vi "WILT Injection Timer 2.vi"(4 "Injection Times":T1, 7 "Station Number in":u32, 8 "Error In":errorcluster, 9 "Current Threshold":dbl=1.0 format="%#_13g", 10 "Step 3 Input":T3, 11 "Dryer Step Pause In":T5 {"Night Cycle Count" format="%04d"; "Day Cycle Count" format="%04d"}) -> (0 "Error Out":errorcluster, 2 "Step 5 Output":T3, 3 "Dryer Step Pause Output":T5 {"Night Cycle Count" format="%04d"; "Day Cycle Count" format="%04d"})   [LabVIEW 2016]
uses:
  Type Definitions/WILT Station Test State Cluster.ctl
  Type Definitions/WILT Dryer Test State.ctl
  Type Definitions/WILT Dryer.ctl
  Type Definitions/WILT Dryer Details.ctl
  Type Definitions/WILT Agilent Channel Definition.ctl
  Type Definitions/WILT DAQ Data.ctl
  Type Definitions/WILT Injection Times.ctl
  Type Definitions/WILT Water Injection Control.ctl
  Globals/WILT Globals Main Program.vi
panel:
  # "Day"
  # "Night"
  # "Day"
  # "Night"
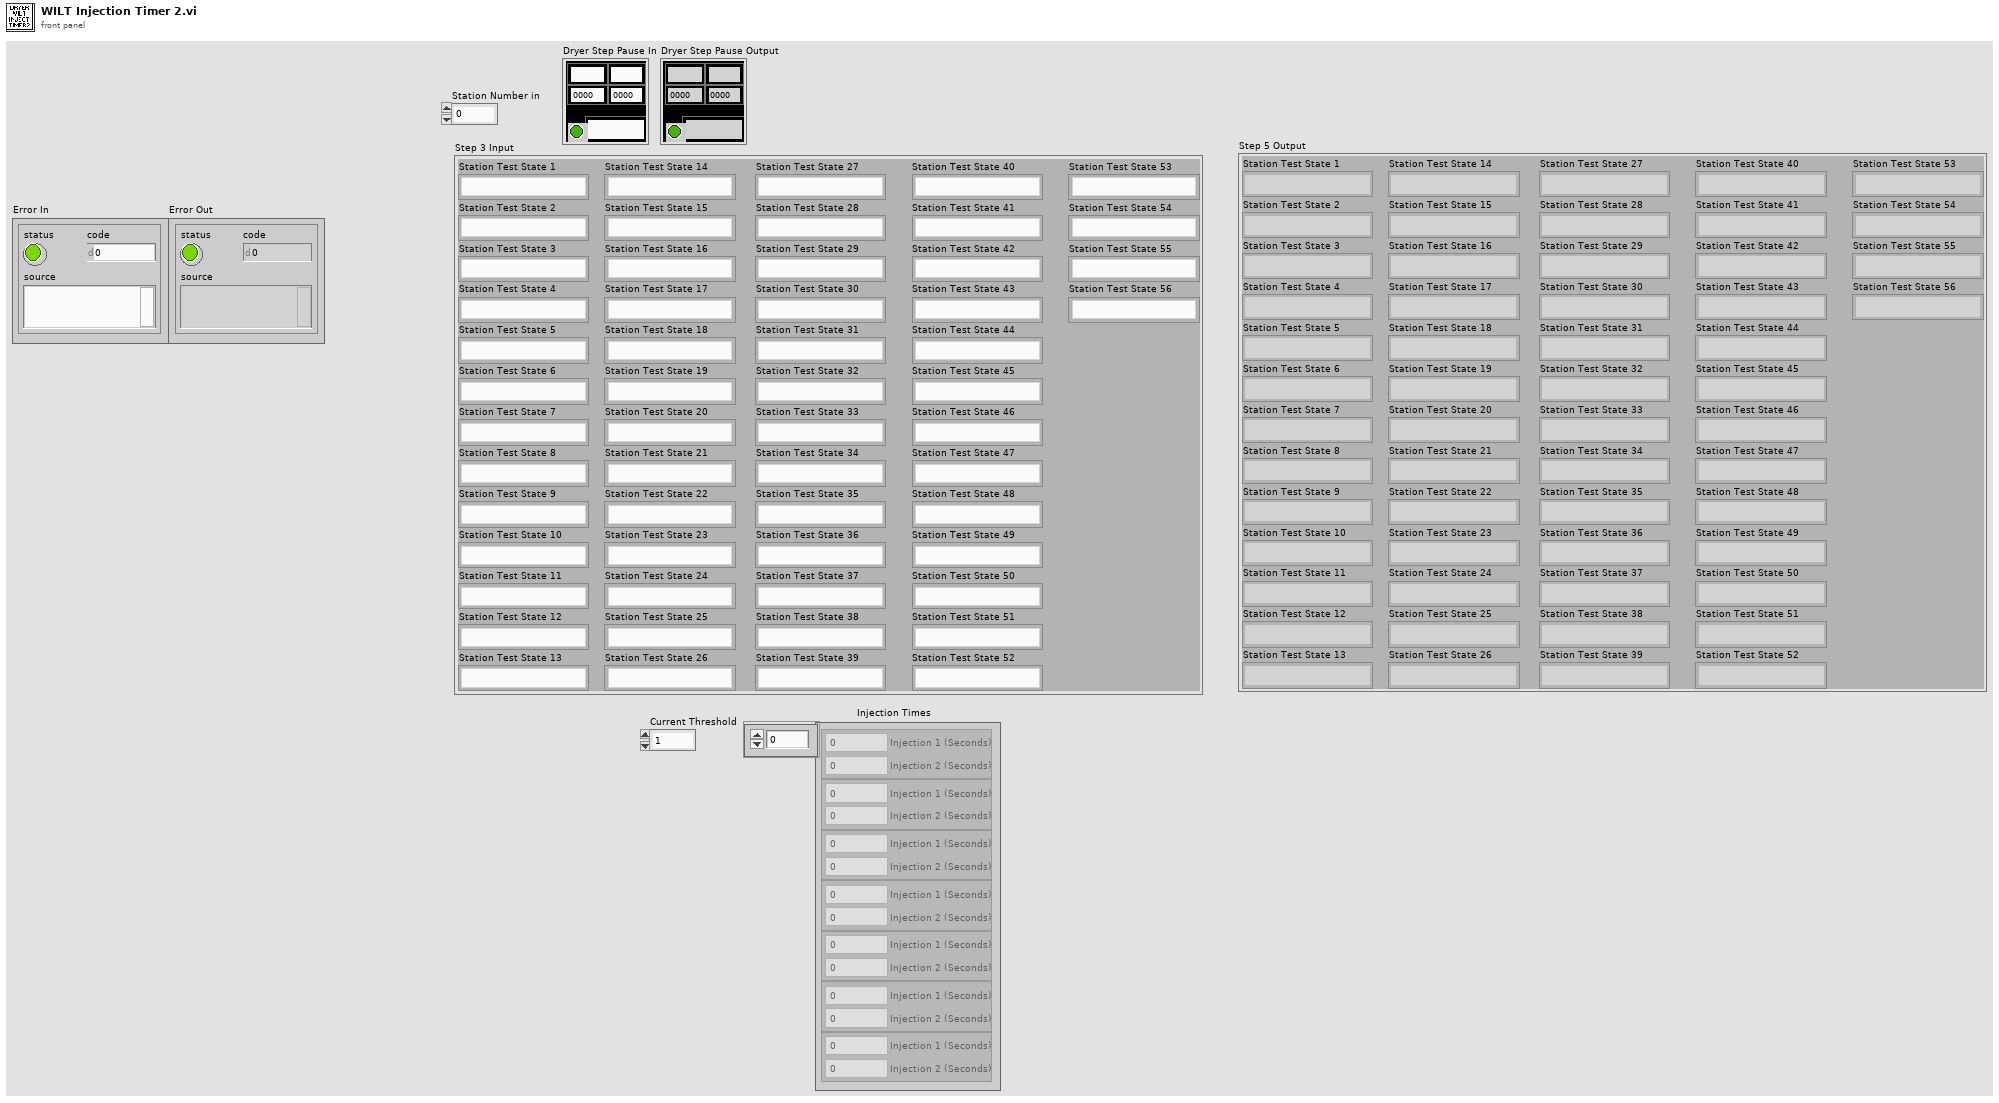
[diagram p1: front panel]
types:
  T1 = typedef "WILT Injection Times.ctl" = T2[]
  T2 = typedef "WILT Water Injection Control.ctl" = cluster{"Injection 1 (Seconds)":dbl, "Injection 2 (Seconds)":dbl}
  T3 = typedef "WILT Station Test State Cluster.ctl" = cluster{"Station Test State 1":T4, "Station Test State 2":T4, "Station Test State 3":T4, "Station Test State 4":T4, "Station Test State 5":T4, "Station Test State 6":T4, "Station Test State 7":T4, "Station Test State 8":T4, "Station Test State 9":T4, "Station Test State 10":T4, "Station Test State 11":T4, "Station Test State 12":T4, "Station Test State 13":T4, "Station Test State 14":T4, "Station Test State 15":T4, "Station Test State 16":T4, "Station Test State 17":T4, "Station Test State 18":T4, "Station Test State 19":T4, "Station Test State 20":T4, "Station Test State 21":T4, "Station Test State 22":T4, "Station Test State 23":T4, "Station Test State 24":T4, "Station Test State 25":T4, "Station Test State 26":T4, "Station Test State 27":T4, "Station Test State 28":T4, "Station Test State 29":T4, "Station Test State 30":T4, "Station Test State 31":T4, "Station Test State 32":T4, "Station Test State 33":T4, "Station Test State 34":T4, "Station Test State 35":T4, "Station Test State 36":T4, "Station Test State 37":T4, "Station Test State 38":T4, "Station Test State 39":T4, "Station Test State 40":T4, "Station Test State 41":T4, "Station Test State 42":T4, "Station Test State 43":T4, "Station Test State 44":T4, "Station Test State 45":T4, "Station Test State 46":T4, "Station Test State 47":T4, "Station Test State 48":T4, "Station Test State 49":T4, "Station Test State 50":T4, "Station Test State 51":T4, "Station Test State 52":T4, "Station Test State 53":T4, "Station Test State 54":T4, "Station Test State 55":T4, "Station Test State 56":T4}
  T4 = typedef "WILT Dryer Test State.ctl" = enum16{"No Serial Number", "Waiting for Dryer To Start", "Drying Clothes", "Water Injection 1 (On)", "Water Injection 1 Timer", "Water Injection 1 (Off)", "Pause Dryer", "Sending Start Stop CMD", "Pause Dryer 2", "Sending Start Stop CMD 2", "Drying Clothes 2", "Water Injection 2 (On)", "Water Injection 2 Timer", "Water Injection 2 (Off)", "Drying Clothes 3", "Cooling Down", "Sending Start Stop CMD 3", "Increment Cycle"}
  T5 = typedef "WILT Dryer.ctl" = cluster{"Lab ID":string, "Day Cycle Count":i32, "Station Label":string, "Dryer Details":T6, "Status Color":u32, "Invisible Button":bool, "Night Cycle Count":i32, "Station Index":i32, "Cycle Index":string, "Audit Alert":bool, "Agilent Channel Definition":T7, "DAQ Data":T8}
  T6 = typedef "WILT Dryer Details.ctl" = cluster{"Station":string, "Lab ID":string, "TR Number":string}
  T7 = typedef "WILT Agilent Channel Definition.ctl" = cluster{"Channel":string, "Station":string, "Label":string, "Agilent Station":string, "Data":dbl}
  T8 = typedef "WILT DAQ Data.ctl" = cluster{"L1 Current":dbl, "L2 Current":dbl, "Temperature  Deg F (TC)":dbl, "Volts":dbl, "Volts (208)":dbl, "SW (208)":dbl}
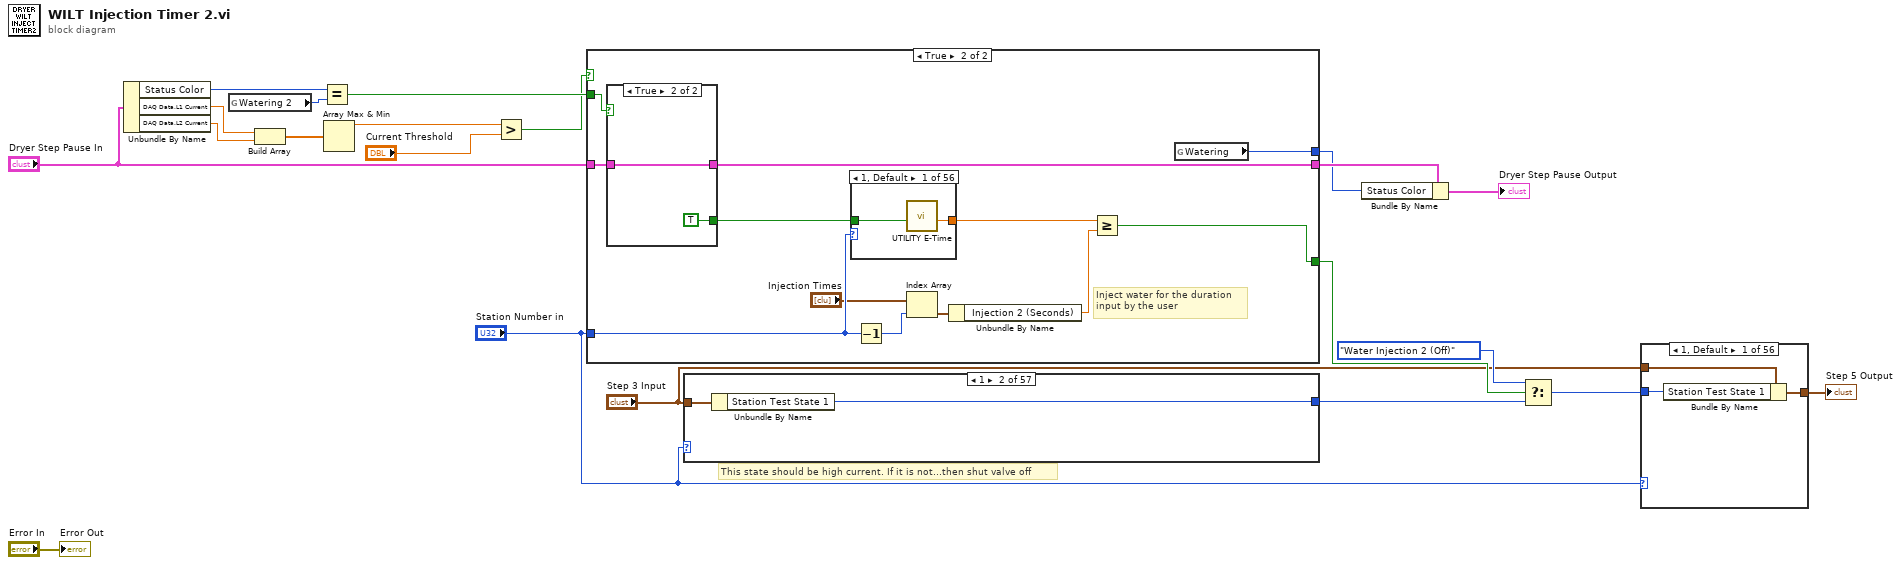
[diagram p0: block diagram]
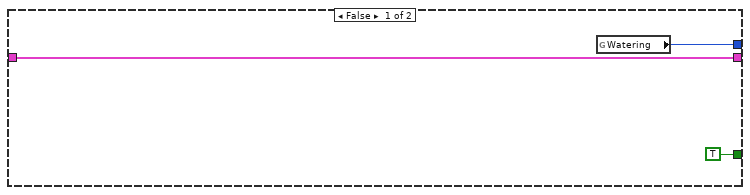
[diagram p2: hidden frame]
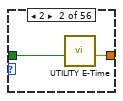
[diagram p3: hidden frame]
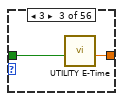
[diagram p4: hidden frame]
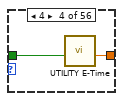
[diagram p5: hidden frame]
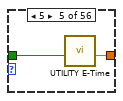
[diagram p6: hidden frame]
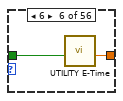
[diagram p7: hidden frame]
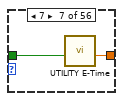
[diagram p8: hidden frame]
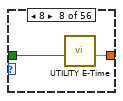
[diagram p9: hidden frame]
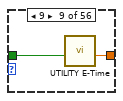
[diagram p10: hidden frame]
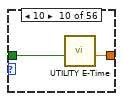
[diagram p11: hidden frame]
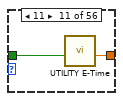
[diagram p12: hidden frame]
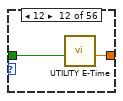
[diagram p13: hidden frame]
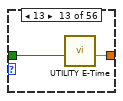
[diagram p14: hidden frame]
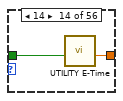
[diagram p15: hidden frame]
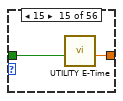
[diagram p16: hidden frame]
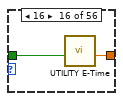
[diagram p17: hidden frame]
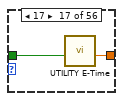
[diagram p18: hidden frame]
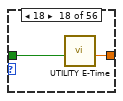
[diagram p19: hidden frame]
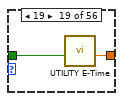
[diagram p20: hidden frame]
diagram:
  # "This state should be high current. If it is not...then shut valve off"
  n1 = Unbundle By Name("Dryer Step Pause In") -> ("Status Color"=w14:u32, "DAQ Data.L1 Current"=w7:dbl, "DAQ Data.L2 Current"=w6:dbl)
  n2 = global read "WILT Globals Main Program.vi" "Watering 2"() -> (w10:u32)
  n3 = Build Array(w7, w6) -> (w5:dbl[])
  n4 = Equal?(x=w14, y=w10) -> (x = y?=w9:bool)
  n5 = Array Max & Min(array=w5) -> (max value=w4:dbl)  [unwired: 3 out]
  n6 = Greater?(x=w4, y="Current Threshold") -> (0:w2:bool)
  n7 = case shown="True" w2 {
    tunnel: [TRUE w36] -> w20
    tunnel: "Dryer Step Pause In" -> [w24 w34]
    tunnel: "Station Number in" -> [_ w33]
    tunnel: w9 -> [_ w30]
    tunnel: [w24 w29] -> w8
    tunnel: [w23 w25] -> w1
    frame False {
      n8 = global read "WILT Globals Main Program.vi" "Watering"() -> (w23:u32)
    }
    frame True {
      # "Inject water for the duration \ninput by the user"
      n9 = case shown="True" w30 {
        tunnel: [FALSE TRUE] -> w28
        tunnel: w34 -> [w149 w151]
        tunnel: [w149 w151] -> w29
        frame False {
        }
        frame True {
        }
      }
      n10 = case shown="1, Default" w33 {
        tunnel: [w38 w39 w41 w43 w45 w47 w49 w51 w53 w55 w57 w59 w61 w63 w65 w67 w69 w71 w73 w75 w77 w79 w81 w83 w85 w87 w89 w91 w93 w95 w97 w99 w101 w103 w105 w107 w109 w111 w113 w115 w117 w119 w121 w123 w125 w127 w129 w131 w133 w135 w137 w139 w141 w143 w145 w147] -> w27
        tunnel: w28 -> [w37 w40 w42 w44 w46 w48 w50 w52 w54 w56 w58 w60 w62 w64 w66 w68 w70 w72 w74 w76 w78 w80 w82 w84 w86 w88 w90 w92 w94 w96 w98 w100 w102 w104 w106 w108 w110 w112 w114 w116 w118 w120 w122 w124 w126 w128 w130 w132 w134 w136 w138 w140 w142 w144 w146 w148]
        frame 1, Default {
          n11 = call "UTILITY E-Time.vi"("Reset"=w37) -> ("Elapsed Time (sec)"=w38:dbl)  [unwired: 8 in, 2 out]
        }
        frame 2 {
          n12 = call "UTILITY E-Time.vi"("Reset"=w40) -> ("Elapsed Time (sec)"=w39:dbl)  [unwired: 8 in, 2 out]
        }
        frame 3 {
          n13 = call "UTILITY E-Time.vi"("Reset"=w42) -> ("Elapsed Time (sec)"=w41:dbl)  [unwired: 8 in, 2 out]
        }
        frame 4 {
          n14 = call "UTILITY E-Time.vi"("Reset"=w44) -> ("Elapsed Time (sec)"=w43:dbl)  [unwired: 8 in, 2 out]
        }
        frame 5 {
          n15 = call "UTILITY E-Time.vi"("Reset"=w46) -> ("Elapsed Time (sec)"=w45:dbl)  [unwired: 8 in, 2 out]
        }
        frame 6 {
          n16 = call "UTILITY E-Time.vi"("Reset"=w48) -> ("Elapsed Time (sec)"=w47:dbl)  [unwired: 8 in, 2 out]
        }
        frame 7 {
          n17 = call "UTILITY E-Time.vi"("Reset"=w50) -> ("Elapsed Time (sec)"=w49:dbl)  [unwired: 8 in, 2 out]
        }
        frame 8 {
          n18 = call "UTILITY E-Time.vi"("Reset"=w52) -> ("Elapsed Time (sec)"=w51:dbl)  [unwired: 8 in, 2 out]
        }
        frame 9 {
          n19 = call "UTILITY E-Time.vi"("Reset"=w54) -> ("Elapsed Time (sec)"=w53:dbl)  [unwired: 8 in, 2 out]
        }
        frame 10 {
          n20 = call "UTILITY E-Time.vi"("Reset"=w56) -> ("Elapsed Time (sec)"=w55:dbl)  [unwired: 8 in, 2 out]
        }
        frame 11 {
          n21 = call "UTILITY E-Time.vi"("Reset"=w58) -> ("Elapsed Time (sec)"=w57:dbl)  [unwired: 8 in, 2 out]
        }
        frame 12 {
          n22 = call "UTILITY E-Time.vi"("Reset"=w60) -> ("Elapsed Time (sec)"=w59:dbl)  [unwired: 8 in, 2 out]
        }
        frame 13 {
          n23 = call "UTILITY E-Time.vi"("Reset"=w62) -> ("Elapsed Time (sec)"=w61:dbl)  [unwired: 8 in, 2 out]
        }
        frame 14 {
          n24 = call "UTILITY E-Time.vi"("Reset"=w64) -> ("Elapsed Time (sec)"=w63:dbl)  [unwired: 8 in, 2 out]
        }
        frame 15 {
          n25 = call "UTILITY E-Time.vi"("Reset"=w66) -> ("Elapsed Time (sec)"=w65:dbl)  [unwired: 8 in, 2 out]
        }
        frame 16 {
          n26 = call "UTILITY E-Time.vi"("Reset"=w68) -> ("Elapsed Time (sec)"=w67:dbl)  [unwired: 8 in, 2 out]
        }
        frame 17 {
          n27 = call "UTILITY E-Time.vi"("Reset"=w70) -> ("Elapsed Time (sec)"=w69:dbl)  [unwired: 8 in, 2 out]
        }
        frame 18 {
          n28 = call "UTILITY E-Time.vi"("Reset"=w72) -> ("Elapsed Time (sec)"=w71:dbl)  [unwired: 8 in, 2 out]
        }
        frame 19 {
          n29 = call "UTILITY E-Time.vi"("Reset"=w74) -> ("Elapsed Time (sec)"=w73:dbl)  [unwired: 8 in, 2 out]
        }
        frame 20 {
          n30 = call "UTILITY E-Time.vi"("Reset"=w76) -> ("Elapsed Time (sec)"=w75:dbl)  [unwired: 8 in, 2 out]
        }
        frame 21 {
          n31 = call "UTILITY E-Time.vi"("Reset"=w78) -> ("Elapsed Time (sec)"=w77:dbl)  [unwired: 8 in, 2 out]
        }
        frame 22 {
          n32 = call "UTILITY E-Time.vi"("Reset"=w80) -> ("Elapsed Time (sec)"=w79:dbl)  [unwired: 8 in, 2 out]
        }
        frame 23 {
          n33 = call "UTILITY E-Time.vi"("Reset"=w82) -> ("Elapsed Time (sec)"=w81:dbl)  [unwired: 8 in, 2 out]
        }
        frame 24 {
          n34 = call "UTILITY E-Time.vi"("Reset"=w84) -> ("Elapsed Time (sec)"=w83:dbl)  [unwired: 8 in, 2 out]
        }
        frame 25 {
          n35 = call "UTILITY E-Time.vi"("Reset"=w86) -> ("Elapsed Time (sec)"=w85:dbl)  [unwired: 8 in, 2 out]
        }
        frame 26 {
          n36 = call "UTILITY E-Time.vi"("Reset"=w88) -> ("Elapsed Time (sec)"=w87:dbl)  [unwired: 8 in, 2 out]
        }
        frame 27 {
          n37 = call "UTILITY E-Time.vi"("Reset"=w90) -> ("Elapsed Time (sec)"=w89:dbl)  [unwired: 8 in, 2 out]
        }
        frame 28 {
          n38 = call "UTILITY E-Time.vi"("Reset"=w92) -> ("Elapsed Time (sec)"=w91:dbl)  [unwired: 8 in, 2 out]
        }
        frame 29 {
          n39 = call "UTILITY E-Time.vi"("Reset"=w94) -> ("Elapsed Time (sec)"=w93:dbl)  [unwired: 8 in, 2 out]
        }
        frame 30 {
          n40 = call "UTILITY E-Time.vi"("Reset"=w96) -> ("Elapsed Time (sec)"=w95:dbl)  [unwired: 8 in, 2 out]
        }
        frame 31 {
          n41 = call "UTILITY E-Time.vi"("Reset"=w98) -> ("Elapsed Time (sec)"=w97:dbl)  [unwired: 8 in, 2 out]
        }
        frame 32 {
          n42 = call "UTILITY E-Time.vi"("Reset"=w100) -> ("Elapsed Time (sec)"=w99:dbl)  [unwired: 8 in, 2 out]
        }
        frame 33 {
          n43 = call "UTILITY E-Time.vi"("Reset"=w102) -> ("Elapsed Time (sec)"=w101:dbl)  [unwired: 8 in, 2 out]
        }
        frame 34 {
          n44 = call "UTILITY E-Time.vi"("Reset"=w104) -> ("Elapsed Time (sec)"=w103:dbl)  [unwired: 8 in, 2 out]
        }
        frame 35 {
          n45 = call "UTILITY E-Time.vi"("Reset"=w106) -> ("Elapsed Time (sec)"=w105:dbl)  [unwired: 8 in, 2 out]
        }
        frame 36 {
          n46 = call "UTILITY E-Time.vi"("Reset"=w108) -> ("Elapsed Time (sec)"=w107:dbl)  [unwired: 8 in, 2 out]
        }
        frame 37 {
          n47 = call "UTILITY E-Time.vi"("Reset"=w110) -> ("Elapsed Time (sec)"=w109:dbl)  [unwired: 8 in, 2 out]
        }
        frame 38 {
          n48 = call "UTILITY E-Time.vi"("Reset"=w112) -> ("Elapsed Time (sec)"=w111:dbl)  [unwired: 8 in, 2 out]
        }
        frame 39 {
          n49 = call "UTILITY E-Time.vi"("Reset"=w114) -> ("Elapsed Time (sec)"=w113:dbl)  [unwired: 8 in, 2 out]
        }
        frame 40 {
          n50 = call "UTILITY E-Time.vi"("Reset"=w116) -> ("Elapsed Time (sec)"=w115:dbl)  [unwired: 8 in, 2 out]
        }
        frame 41 {
          n51 = call "UTILITY E-Time.vi"("Reset"=w118) -> ("Elapsed Time (sec)"=w117:dbl)  [unwired: 8 in, 2 out]
        }
        frame 42 {
          n52 = call "UTILITY E-Time.vi"("Reset"=w120) -> ("Elapsed Time (sec)"=w119:dbl)  [unwired: 8 in, 2 out]
        }
        frame 43 {
          n53 = call "UTILITY E-Time.vi"("Reset"=w122) -> ("Elapsed Time (sec)"=w121:dbl)  [unwired: 8 in, 2 out]
        }
        frame 44 {
          n54 = call "UTILITY E-Time.vi"("Reset"=w124) -> ("Elapsed Time (sec)"=w123:dbl)  [unwired: 8 in, 2 out]
        }
        frame 45 {
          n55 = call "UTILITY E-Time.vi"("Reset"=w126) -> ("Elapsed Time (sec)"=w125:dbl)  [unwired: 8 in, 2 out]
        }
        frame 46 {
          n56 = call "UTILITY E-Time.vi"("Reset"=w128) -> ("Elapsed Time (sec)"=w127:dbl)  [unwired: 8 in, 2 out]
        }
        frame 47 {
          n57 = call "UTILITY E-Time.vi"("Reset"=w130) -> ("Elapsed Time (sec)"=w129:dbl)  [unwired: 8 in, 2 out]
        }
        frame 48 {
          n58 = call "UTILITY E-Time.vi"("Reset"=w132) -> ("Elapsed Time (sec)"=w131:dbl)  [unwired: 8 in, 2 out]
        }
        frame 49 {
          n59 = call "UTILITY E-Time.vi"("Reset"=w134) -> ("Elapsed Time (sec)"=w133:dbl)  [unwired: 8 in, 2 out]
        }
        frame 50 {
          n60 = call "UTILITY E-Time.vi"("Reset"=w136) -> ("Elapsed Time (sec)"=w135:dbl)  [unwired: 8 in, 2 out]
        }
        frame 51 {
          n61 = call "UTILITY E-Time.vi"("Reset"=w138) -> ("Elapsed Time (sec)"=w137:dbl)  [unwired: 8 in, 2 out]
        }
        frame 52 {
          n62 = call "UTILITY E-Time.vi"("Reset"=w140) -> ("Elapsed Time (sec)"=w139:dbl)  [unwired: 8 in, 2 out]
        }
        frame 53 {
          n63 = call "UTILITY E-Time.vi"("Reset"=w142) -> ("Elapsed Time (sec)"=w141:dbl)  [unwired: 8 in, 2 out]
        }
        frame 54 {
          n64 = call "UTILITY E-Time.vi"("Reset"=w144) -> ("Elapsed Time (sec)"=w143:dbl)  [unwired: 8 in, 2 out]
        }
        frame 55 {
          n65 = call "UTILITY E-Time.vi"("Reset"=w146) -> ("Elapsed Time (sec)"=w145:dbl)  [unwired: 8 in, 2 out]
        }
        frame 56 {
          n66 = call "UTILITY E-Time.vi"("Reset"=w148) -> ("Elapsed Time (sec)"=w147:dbl)  [unwired: 8 in, 2 out]
        }
      }
      n67 = Decrement(x=w33) -> (x-1=w35:u32)
      n68 = Index Array(array="Injection Times", index=w35) -> (element=w32:T2)
      n69 = Unbundle By Name(w32) -> ("Injection 2 (Seconds)"=w31:dbl)
      n70 = Greater Or Equal?(x=w27, y=w31) -> (x >= y?=w36:bool)
      n71 = global read "WILT Globals Main Program.vi" "Watering"() -> (w25:u32)
    }
  }
  n72 = case shown="1" "Station Number in" {
    tunnel: "Step 3 Input" -> [_ w155 w157 w159 w161 w163 w165 w167 w169 w171 w173 w175 w177 w179 w181 w183 w185 w187 w189 w191 w193 w195 w197 w199 w201 w203 w205 w207 w209 w211 w213 w215 w217 w219 w221 w223 w225 w227 w229 w231 w233 w235 w237 w239 w241 w243 w245 w247 w249 w251 w253 w255 w257 w259 w261 w263 w265]
    tunnel: [WILT_Dryer_Test_State."No Serial Number" ("Station Test State 56") w154 w156 w158 w160 w162 w164 w166 w168 w170 w172 w174 w176 w178 w180 w182 w184 w186 w188 w190 w192 w194 w196 w198 w200 w202 w204 w206 w208 w210 w212 w214 w216 w218 w220 w222 w224 w226 w228 w230 w232 w234 w236 w238 w240 w242 w244 w246 w248 w250 w252 w254 w256 w258 w260 w262 w264] -> w16
    frame 0, Default {
      # "This is not a station.\nDo nothing"
    }
    frame 1 {
      n73 = Unbundle By Name(w155) -> ("Station Test State 1"=w154:T4)
    }
    frame 2 {
      n74 = Unbundle By Name(w157) -> ("Station Test State 2"=w156:T4)
    }
    frame 3 {
      n75 = Unbundle By Name(w159) -> ("Station Test State 3"=w158:T4)
    }
    frame 4 {
      n76 = Unbundle By Name(w161) -> ("Station Test State 4"=w160:T4)
    }
    frame 5 {
      n77 = Unbundle By Name(w163) -> ("Station Test State 5"=w162:T4)
    }
    frame 6 {
      n78 = Unbundle By Name(w165) -> ("Station Test State 6"=w164:T4)
    }
    frame 7 {
      n79 = Unbundle By Name(w167) -> ("Station Test State 7"=w166:T4)
    }
    frame 8 {
      n80 = Unbundle By Name(w169) -> ("Station Test State 8"=w168:T4)
    }
    frame 9 {
      n81 = Unbundle By Name(w171) -> ("Station Test State 9"=w170:T4)
    }
    frame 10 {
      n82 = Unbundle By Name(w173) -> ("Station Test State 10"=w172:T4)
    }
    frame 11 {
      n83 = Unbundle By Name(w175) -> ("Station Test State 11"=w174:T4)
    }
    frame 12 {
      n84 = Unbundle By Name(w177) -> ("Station Test State 12"=w176:T4)
    }
    frame 13 {
      n85 = Unbundle By Name(w179) -> ("Station Test State 13"=w178:T4)
    }
    frame 14 {
      n86 = Unbundle By Name(w181) -> ("Station Test State 14"=w180:T4)
    }
    frame 15 {
      n87 = Unbundle By Name(w183) -> ("Station Test State 15"=w182:T4)
    }
    frame 16 {
      n88 = Unbundle By Name(w185) -> ("Station Test State 16"=w184:T4)
    }
    frame 17 {
      n89 = Unbundle By Name(w187) -> ("Station Test State 17"=w186:T4)
    }
    frame 18 {
      n90 = Unbundle By Name(w189) -> ("Station Test State 18"=w188:T4)
    }
    frame 19 {
      n91 = Unbundle By Name(w191) -> ("Station Test State 19"=w190:T4)
    }
    frame 20 {
      n92 = Unbundle By Name(w193) -> ("Station Test State 20"=w192:T4)
    }
    frame 21 {
      n93 = Unbundle By Name(w195) -> ("Station Test State 21"=w194:T4)
    }
    frame 22 {
      n94 = Unbundle By Name(w197) -> ("Station Test State 22"=w196:T4)
    }
    frame 23 {
      n95 = Unbundle By Name(w199) -> ("Station Test State 23"=w198:T4)
    }
    frame 24 {
      n96 = Unbundle By Name(w201) -> ("Station Test State 24"=w200:T4)
    }
    frame 25 {
      n97 = Unbundle By Name(w203) -> ("Station Test State 25"=w202:T4)
    }
    frame 26 {
      n98 = Unbundle By Name(w205) -> ("Station Test State 26"=w204:T4)
    }
    frame 27 {
      n99 = Unbundle By Name(w207) -> ("Station Test State 27"=w206:T4)
    }
    frame 28 {
      n100 = Unbundle By Name(w209) -> ("Station Test State 28"=w208:T4)
    }
    frame 29 {
      n101 = Unbundle By Name(w211) -> ("Station Test State 29"=w210:T4)
    }
    frame 30 {
      n102 = Unbundle By Name(w213) -> ("Station Test State 30"=w212:T4)
    }
    frame 31 {
      n103 = Unbundle By Name(w215) -> ("Station Test State 31"=w214:T4)
    }
    frame 32 {
      n104 = Unbundle By Name(w217) -> ("Station Test State 32"=w216:T4)
    }
    frame 33 {
      n105 = Unbundle By Name(w219) -> ("Station Test State 33"=w218:T4)
    }
    frame 34 {
      n106 = Unbundle By Name(w221) -> ("Station Test State 34"=w220:T4)
    }
    frame 35 {
      n107 = Unbundle By Name(w223) -> ("Station Test State 35"=w222:T4)
    }
    frame 36 {
      n108 = Unbundle By Name(w225) -> ("Station Test State 36"=w224:T4)
    }
    frame 37 {
      n109 = Unbundle By Name(w227) -> ("Station Test State 37"=w226:T4)
    }
    frame 38 {
      n110 = Unbundle By Name(w229) -> ("Station Test State 38"=w228:T4)
    }
    frame 39 {
      n111 = Unbundle By Name(w231) -> ("Station Test State 39"=w230:T4)
    }
    frame 40 {
      n112 = Unbundle By Name(w233) -> ("Station Test State 40"=w232:T4)
    }
    frame 41 {
      n113 = Unbundle By Name(w235) -> ("Station Test State 41"=w234:T4)
    }
    frame 42 {
      n114 = Unbundle By Name(w237) -> ("Station Test State 42"=w236:T4)
    }
    frame 43 {
      n115 = Unbundle By Name(w239) -> ("Station Test State 43"=w238:T4)
    }
    frame 44 {
      n116 = Unbundle By Name(w241) -> ("Station Test State 44"=w240:T4)
    }
    frame 45 {
      n117 = Unbundle By Name(w243) -> ("Station Test State 45"=w242:T4)
    }
    frame 46 {
      n118 = Unbundle By Name(w245) -> ("Station Test State 46"=w244:T4)
    }
    frame 47 {
      n119 = Unbundle By Name(w247) -> ("Station Test State 47"=w246:T4)
    }
    frame 48 {
      n120 = Unbundle By Name(w249) -> ("Station Test State 48"=w248:T4)
    }
    frame 49 {
      n121 = Unbundle By Name(w251) -> ("Station Test State 49"=w250:T4)
    }
    frame 50 {
      n122 = Unbundle By Name(w253) -> ("Station Test State 50"=w252:T4)
    }
    frame 51 {
      n123 = Unbundle By Name(w255) -> ("Station Test State 51"=w254:T4)
    }
    frame 52 {
      n124 = Unbundle By Name(w257) -> ("Station Test State 52"=w256:T4)
    }
    frame 53 {
      n125 = Unbundle By Name(w259) -> ("Station Test State 53"=w258:T4)
    }
    frame 54 {
      n126 = Unbundle By Name(w261) -> ("Station Test State 54"=w260:T4)
    }
    frame 55 {
      n127 = Unbundle By Name(w263) -> ("Station Test State 55"=w262:T4)
    }
    frame 56 {
      n128 = Unbundle By Name(w265) -> ("Station Test State 56"=w264:T4)
    }
  }
  n129 = Bundle By Name(cluster=w8, "Status Color"=w1) -> (→"Dryer Step Pause Output":T5)
  n130 = Select(t=WILT_Dryer_Test_State."Water Injection 2 (Off)" ("Current State 2"), s=w20, f=w16) -> (s? t:f=w15:T4)
  n131 = case shown="1, Default" "Station Number in" {
    tunnel: "Step 3 Input" -> [w268 w271 w274 w277 w280 w283 w286 w289 w292 w295 w298 w301 w304 w307 w310 w313 w316 w319 w322 w325 w328 w331 w334 w337 w340 w343 w346 w349 w352 w355 w358 w361 w364 w367 w370 w373 w376 w379 w382 w385 w388 w391 w394 w397 w400 w403 w406 w409 w412 w415 w418 w421 w424 w427 w430 w433]
    tunnel: w15 -> [w267 w269 w272 w275 w278 w281 w284 w287 w290 w293 w296 w299 w302 w305 w308 w311 w314 w317 w320 w323 w326 w329 w332 w335 w338 w341 w344 w347 w350 w353 w356 w359 w362 w365 w368 w371 w374 w377 w380 w383 w386 w389 w392 w395 w398 w401 w404 w407 w410 w413 w416 w419 w422 w425 w428 w431]
    tunnel: [w266 w270 w273 w276 w279 w282 w285 w288 w291 w294 w297 w300 w303 w306 w309 w312 w315 w318 w321 w324 w327 w330 w333 w336 w339 w342 w345 w348 w351 w354 w357 w360 w363 w366 w369 w372 w375 w378 w381 w384 w387 w390 w393 w396 w399 w402 w405 w408 w411 w414 w417 w420 w423 w426 w429 w432] -> w18
    frame 1, Default {
      n132 = Bundle By Name(cluster=w268, "Station Test State 1"=w267) -> (w266:T3)
    }
    frame 2 {
      n133 = Bundle By Name(cluster=w271, "Station Test State 2"=w269) -> (w270:T3)
    }
    frame 3 {
      n134 = Bundle By Name(cluster=w274, "Station Test State 3"=w272) -> (w273:T3)
    }
    frame 4 {
      n135 = Bundle By Name(cluster=w277, "Station Test State 4"=w275) -> (w276:T3)
    }
    frame 5 {
      n136 = Bundle By Name(cluster=w280, "Station Test State 5"=w278) -> (w279:T3)
    }
    frame 6 {
      n137 = Bundle By Name(cluster=w283, "Station Test State 6"=w281) -> (w282:T3)
    }
    frame 7 {
      n138 = Bundle By Name(cluster=w286, "Station Test State 7"=w284) -> (w285:T3)
    }
    frame 8 {
      n139 = Bundle By Name(cluster=w289, "Station Test State 8"=w287) -> (w288:T3)
    }
    frame 9 {
      n140 = Bundle By Name(cluster=w292, "Station Test State 9"=w290) -> (w291:T3)
    }
    frame 10 {
      n141 = Bundle By Name(cluster=w295, "Station Test State 10"=w293) -> (w294:T3)
    }
    frame 11 {
      n142 = Bundle By Name(cluster=w298, "Station Test State 11"=w296) -> (w297:T3)
    }
    frame 12 {
      n143 = Bundle By Name(cluster=w301, "Station Test State 12"=w299) -> (w300:T3)
    }
    frame 13 {
      n144 = Bundle By Name(cluster=w304, "Station Test State 13"=w302) -> (w303:T3)
    }
    frame 14 {
      n145 = Bundle By Name(cluster=w307, "Station Test State 14"=w305) -> (w306:T3)
    }
    frame 15 {
      n146 = Bundle By Name(cluster=w310, "Station Test State 15"=w308) -> (w309:T3)
    }
    frame 16 {
      n147 = Bundle By Name(cluster=w313, "Station Test State 16"=w311) -> (w312:T3)
    }
    frame 17 {
      n148 = Bundle By Name(cluster=w316, "Station Test State 17"=w314) -> (w315:T3)
    }
    frame 18 {
      n149 = Bundle By Name(cluster=w319, "Station Test State 18"=w317) -> (w318:T3)
    }
    frame 19 {
      n150 = Bundle By Name(cluster=w322, "Station Test State 19"=w320) -> (w321:T3)
    }
    frame 20 {
      n151 = Bundle By Name(cluster=w325, "Station Test State 20"=w323) -> (w324:T3)
    }
    frame 21 {
      n152 = Bundle By Name(cluster=w328, "Station Test State 21"=w326) -> (w327:T3)
    }
    frame 22 {
      n153 = Bundle By Name(cluster=w331, "Station Test State 22"=w329) -> (w330:T3)
    }
    frame 23 {
      n154 = Bundle By Name(cluster=w334, "Station Test State 23"=w332) -> (w333:T3)
    }
    frame 24 {
      n155 = Bundle By Name(cluster=w337, "Station Test State 24"=w335) -> (w336:T3)
    }
    frame 25 {
      n156 = Bundle By Name(cluster=w340, "Station Test State 25"=w338) -> (w339:T3)
    }
    frame 26 {
      n157 = Bundle By Name(cluster=w343, "Station Test State 26"=w341) -> (w342:T3)
    }
    frame 27 {
      n158 = Bundle By Name(cluster=w346, "Station Test State 27"=w344) -> (w345:T3)
    }
    frame 28 {
      n159 = Bundle By Name(cluster=w349, "Station Test State 28"=w347) -> (w348:T3)
    }
    frame 29 {
      n160 = Bundle By Name(cluster=w352, "Station Test State 29"=w350) -> (w351:T3)
    }
    frame 30 {
      n161 = Bundle By Name(cluster=w355, "Station Test State 30"=w353) -> (w354:T3)
    }
    frame 31 {
      n162 = Bundle By Name(cluster=w358, "Station Test State 31"=w356) -> (w357:T3)
    }
    frame 32 {
      n163 = Bundle By Name(cluster=w361, "Station Test State 32"=w359) -> (w360:T3)
    }
    frame 33 {
      n164 = Bundle By Name(cluster=w364, "Station Test State 33"=w362) -> (w363:T3)
    }
    frame 34 {
      n165 = Bundle By Name(cluster=w367, "Station Test State 34"=w365) -> (w366:T3)
    }
    frame 35 {
      n166 = Bundle By Name(cluster=w370, "Station Test State 35"=w368) -> (w369:T3)
    }
    frame 36 {
      n167 = Bundle By Name(cluster=w373, "Station Test State 36"=w371) -> (w372:T3)
    }
    frame 37 {
      n168 = Bundle By Name(cluster=w376, "Station Test State 37"=w374) -> (w375:T3)
    }
    frame 38 {
      n169 = Bundle By Name(cluster=w379, "Station Test State 38"=w377) -> (w378:T3)
    }
    frame 39 {
      n170 = Bundle By Name(cluster=w382, "Station Test State 39"=w380) -> (w381:T3)
    }
    frame 40 {
      n171 = Bundle By Name(cluster=w385, "Station Test State 40"=w383) -> (w384:T3)
    }
    frame 41 {
      n172 = Bundle By Name(cluster=w388, "Station Test State 41"=w386) -> (w387:T3)
    }
    frame 42 {
      n173 = Bundle By Name(cluster=w391, "Station Test State 42"=w389) -> (w390:T3)
    }
    frame 43 {
      n174 = Bundle By Name(cluster=w394, "Station Test State 43"=w392) -> (w393:T3)
    }
    frame 44 {
      n175 = Bundle By Name(cluster=w397, "Station Test State 44"=w395) -> (w396:T3)
    }
    frame 45 {
      n176 = Bundle By Name(cluster=w400, "Station Test State 45"=w398) -> (w399:T3)
    }
    frame 46 {
      n177 = Bundle By Name(cluster=w403, "Station Test State 46"=w401) -> (w402:T3)
    }
    frame 47 {
      n178 = Bundle By Name(cluster=w406, "Station Test State 47"=w404) -> (w405:T3)
    }
    frame 48 {
      n179 = Bundle By Name(cluster=w409, "Station Test State 48"=w407) -> (w408:T3)
    }
    frame 49 {
      n180 = Bundle By Name(cluster=w412, "Station Test State 49"=w410) -> (w411:T3)
    }
    frame 50 {
      n181 = Bundle By Name(cluster=w415, "Station Test State 50"=w413) -> (w414:T3)
    }
    frame 51 {
      n182 = Bundle By Name(cluster=w418, "Station Test State 51"=w416) -> (w417:T3)
    }
    frame 52 {
      n183 = Bundle By Name(cluster=w421, "Station Test State 52"=w419) -> (w420:T3)
    }
    frame 53 {
      n184 = Bundle By Name(cluster=w424, "Station Test State 53"=w422) -> (w423:T3)
    }
    frame 54 {
      n185 = Bundle By Name(cluster=w427, "Station Test State 54"=w425) -> (w426:T3)
    }
    frame 55 {
      n186 = Bundle By Name(cluster=w430, "Station Test State 55"=w428) -> (w429:T3)
    }
    frame 56 {
      n187 = Bundle By Name(cluster=w433, "Station Test State 56"=w431) -> (w432:T3)
    }
  }
  "Step 5 Output" <- w18
  "Error Out" <- "Error In"
